vi "BRig_dataLC_Reward_Block_l1.vi"() -> (2 "output_Reward_Block":i32)   [LabVIEW 2014]
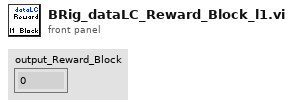
[diagram p1: front panel]
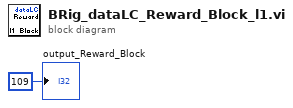
[diagram p0: block diagram]
diagram:
  "output_Reward_Block" <- 109 ("output_iBlock")
